vi "ep_Get Significance (ICM).vi"(0 "spectra points in window":T4(array[cluster]), 1 "pole pairs":i32, 2 "fundamental frequency [Hz]":dbl, 5 "peaks information":T3(array[cluster]), 7 "enough points for peak search?":bool[](array[boolean]), 9 "number of peaks":i32[](array[numeric]), 11 "error in (no error)":errorcluster, 12 "minimum max-magnitude":dbl, 13 "range of speed":T1) -> (4 "top3 speed data":cluster{"speed [RPM]":dbl, "slip":dbl}[](array[cluster]), 6 "top3 significance":dbl[](array[numeric]), 8 "top3 harmonic for speed calculation":T2[](array[typedef]), 14 "candidate speeds":cluster{"speed [RPM]":dbl, "slip":dbl}[](array[cluster]), 15 "error out":errorcluster)   [LabVIEW 2017]
uses:
  <vilib>/addons/Electrical Power/Motor Monitoring/subVIs/ep_Harmonic for Speed Calculation.ctl
  <vilib>/Analysis/baseanly.llb/Mean (DBL).vi
  <vilib>/Analysis/NI_AALBase.lvlib
  <vilib>/addons/Electrical Power/Motor Monitoring/NI_EP_Motor Monitoring.lvlib
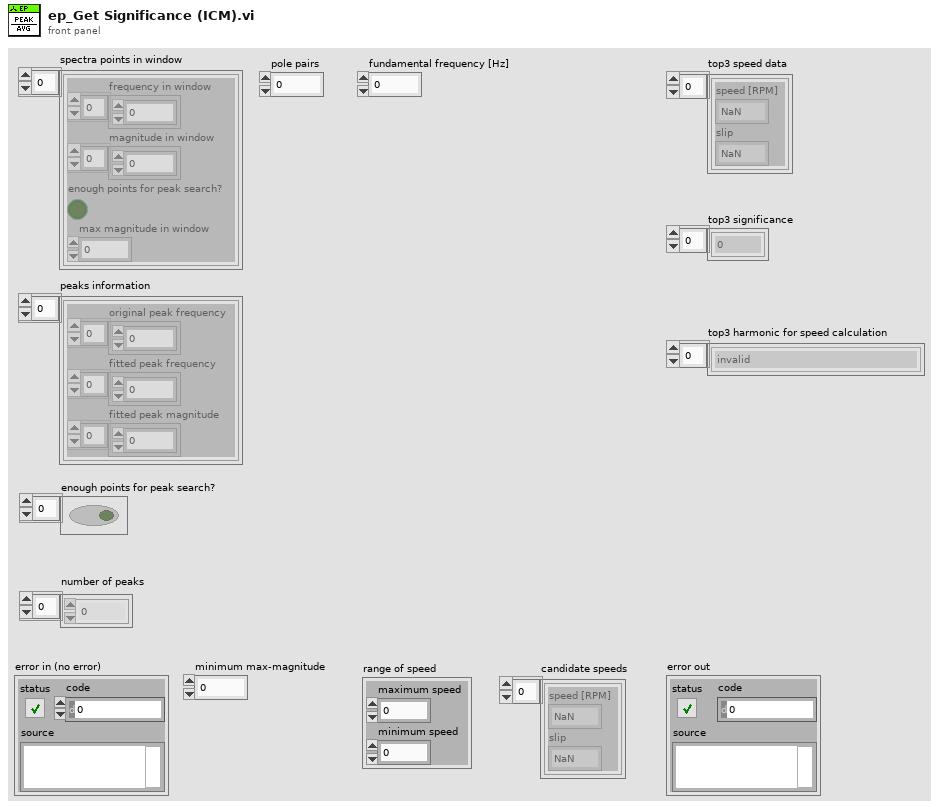
[diagram p1: front panel]
types:
  T1 = cluster{"maximum speed":dbl, "minimum speed":dbl}
  T2 = typedef "NI_EP_Motor Monitoring.lvlib/ep_Harmonic for Speed Calculation.ctl" = enum16{"invalid", "fr", "2fs-2fr", "2fs-fr", "2fr"}
  T3 = cluster{"original peak frequency":dbl[], "fitted peak frequency":dbl[], "fitted peak magnitude":dbl[]}[]
  T4 = cluster{"frequency in window":dbl[], "magnitude in window":dbl[], "enough points for peak search?":bool, "max magnitude in window":dbl}[]
  T5 = typedef "NI_EP_Motor Monitoring.lvlib/ep_Case for Speed Calculation.ctl" = enum16{"no available harmonic for speed calculation", "use the harmonic with highest magnitude", "use the harmonic with highest significance"}
  T6 = cluster{"frequency in window":dbl[], "magnitude in window":dbl[], "enough points for peak search?":bool, "max magnitude in window":dbl}
  T7 = cluster{"maximum frequency [Hz]":dbl, "slip error allowance":dbl, "minimum points for peak search":dbl, "accuracy of fs":dbl, "difference?":bool, " fs harmonics order":i32, "fs forbidden range":dbl, "p3:p1 valid significance ratio":dbl, "ratio for significance weighting":dbl, "significance weighting":dbl}
  T8 = cluster{"original peak frequency":dbl[], "fitted peak frequency":dbl[], "fitted peak magnitude":dbl[]}
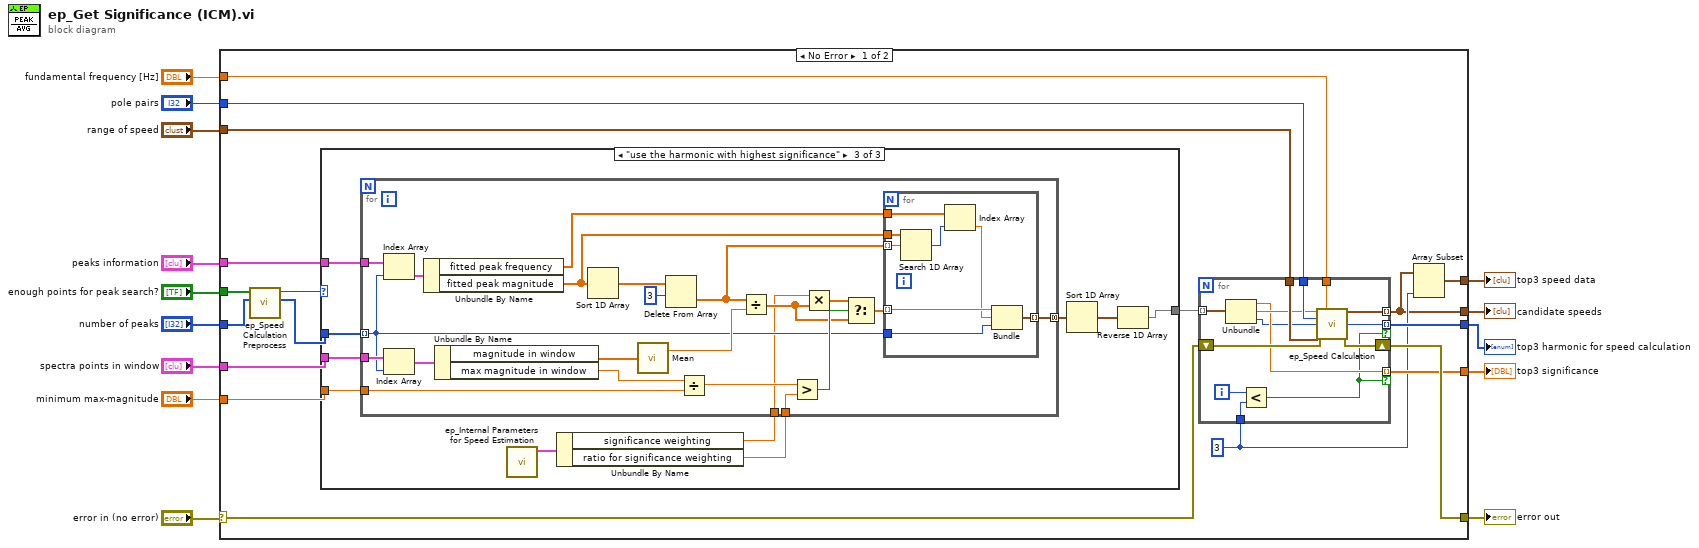
[diagram p0: block diagram]
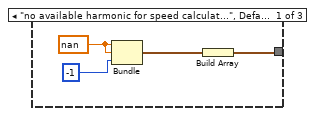
[diagram p2: hidden frame]
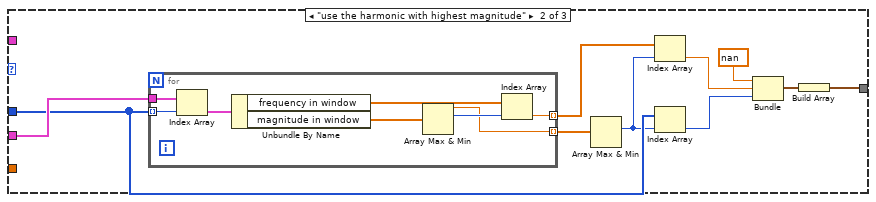
[diagram p3: hidden frame]
diagram:
  n1 = case shown="No Error" "error in (no error)" {
    selector: "error in (no error)" -> [w29 w109]
    tunnel: [w28 w109] -> w13
    tunnel: "peaks information" -> [w32 _]
    tunnel: "spectra points in window" -> [w30 _]
    tunnel: [w31 _] -> w10
    tunnel: [w16 _] -> w9
    tunnel: "fundamental frequency [Hz]" -> [w27 _]
    tunnel: "pole pairs" -> [w26 _]
    tunnel: "range of speed" -> [w25 _]
    tunnel: [w23 _] -> w5
    tunnel: "minimum max-magnitude" -> [w22 _]
    tunnel: "enough points for peak search?" -> [w19 _]
    tunnel: "number of peaks" -> [w18 _]
    tunnel: [w15 _] -> w1
    frame No Error {
      w17 = 3 ("y")
      n2 = call <vilib>:"ep_Speed Calculation Preprocess.vi"("number of peaks"=w18, "enough points for peak search?"=w19) -> ("harmonic for comparison"=w20:i32[], "case for speed calculation"=w21:T5)  [unwired: 8 in]
      n3 = case shown="\"use the harmonic with highest significance\"" w21 {
        tunnel: w32 -> [_ _ w78]
        tunnel: w30 -> [_ w60 w76]
        tunnel: w20 -> [_ w58 w77]
        tunnel: [w47 w54 w74] -> w24
        tunnel: w22 -> [_ _ w72]
        frame "no available harmonic for speed calculation", Default {
          w50 = nan
          n4 = Bundle(w50, w50, -1) -> (w48:cluster{dbl, dbl, i32})  [unwired: 1 in]
          n5 = Build Array(w48) -> (w47:cluster{dbl, dbl, i32}[])
        }
        frame "use the harmonic with highest magnitude" {
          n6 = for {
            tunnel: w58 -> [w67] mode=indexing
            tunnel: w60 -> [w68]
            tunnel: [w62] -> w59 mode=indexing
            tunnel: [w61] -> w57 mode=indexing
            n7 = Index Array(array=w68, index=w67) -> (element=w66:T6)
            n8 = Unbundle By Name(w66) -> ("frequency in window"=w64:dbl[], "magnitude in window"=w65:dbl[])
            n9 = Array Max & Min(array=w65) -> (max value=w62:dbl, max index (indices)=w63:i32)  [unwired: 2 out]
            n10 = Index Array(array=w64, index=w63) -> (element=w61:dbl)
          }
          n11 = Array Max & Min(array=w59) -> (max index (indices)=w56:i32)  [unwired: 3 out]
          n12 = Index Array(array=w57, index=w56) -> (element=w52:dbl)
          n13 = Index Array(array=w58, index=w56) -> (element=w51:i32)
          n14 = Bundle(nan, "frequency points"=w52, w51) -> (w53:cluster{dbl, "frequency points":dbl, i32})  [unwired: 1 in]
          n15 = Build Array(w53) -> (w54:cluster{dbl, "frequency points":dbl, i32}[])
        }
        frame "use the harmonic with highest significance" {
          n16 = call <vilib>:"ep_Internal Parameters for Speed Estimation.vi"() -> ("internal parameters for speed estimation"=w73:T7)  [unwired: 11 in]
          n17 = Unbundle By Name(w73) -> ("significance weighting"=w70:dbl, "ratio for significance weighting"=w71:dbl)
          n18 = for {
            tunnel: w78 -> [w100]
            tunnel: w77 -> [w87] mode=indexing
            tunnel: w76 -> [w97]
            tunnel: [w86] -> w75 mode=concatenating
            tunnel: w72 -> [w81]
            tunnel: w71 -> [w80]
            tunnel: w70 -> [w79]
            n19 = Index Array(array=w100, index=w87) -> (element=w98:T8)
            n20 = Index Array(array=w97, index=w87) -> (element=w92:T6)
            n21 = Unbundle By Name(w98) -> ("fitted peak frequency"=w99:dbl[], "fitted peak magnitude"=w96:dbl[])
            n22 = Unbundle By Name(w92) -> ("magnitude in window"=w91:dbl[], "max magnitude in window"=w82:dbl)
            n23 = Sort 1D Array(array=w96) -> (sorted array=w85:dbl[])
            n24 = call-poly <vilib>:"Mean.vi"("X"=w91) -> ("mean"=w93:dbl)  [unwired: 1 out]
            n25 = Delete From Array(array=w85, length=3 ("index")) -> (deleted portion=w83:dbl[])  [unwired: 1 in, 1 out]
            n26 = Divide(x=w82, y=w81) -> (x/y=w95:dbl)
            n27 = Divide(x=w83, y=w93) -> (x/y=w89:dbl[])
            n28 = Greater?(x=w95, y=w80) -> (0:w94:bool)
            n29 = Multiply(x=w79, y=w89) -> (x*y=w90:dbl[])
            n30 = Select(t=w90, s=w94, f=w89) -> (s? t:f=w88:dbl[])
            n31 = for {
              tunnel: w99 -> [w107]
              tunnel: w83 -> [w108] mode=indexing
              tunnel: w96 -> [w106]
              tunnel: w88 -> [w102] mode=indexing
              tunnel: w87 -> [w104]
              tunnel: [w103] -> w86 mode=indexing
              n32 = Search 1D Array(1D array=w106, element=w108) -> (index of element=w105:i32)  [unwired: 1 in]
              n33 = Index Array(array=w107, index=w105) -> (element=w101:dbl)
              n34 = Bundle(w102, w101, w104) -> (w103:cluster{dbl, dbl, i32})  [unwired: 1 in]
            }
          }
          n35 = Sort 1D Array(array=w75) -> (sorted array=w69:cluster{dbl, dbl, i32}[])
          n36 = Reverse 1D Array(array=w69) -> (reversed array=w74:cluster{dbl, dbl, i32}[])
        }
      }
      n37 = for {
        tunnel: [w36] -> w31 mode=indexing if=w34
        shift-right: [w45] -> w28
        shift-left: w29 -> [w46]
        tunnel: [w44] -> w15 mode=indexing
        tunnel: w27 -> [w43]
        tunnel: w26 -> [w42]
        tunnel: w25 -> [w41]
        tunnel: w24 -> [w40] mode=indexing
        tunnel: [w38] -> w23 mode=indexing if=w34
        tunnel: w17 -> [w33]
        i -> [w35]
        n38 = Unbundle(w40) -> (w38:dbl, "frequency points"=w39:dbl, w37:i32)
        n39 = Less?(x=w35, y=w33) -> (x < y?=w34:bool)
        n40 = call <vilib>:"ep_Speed Calculation.vi"("harmonic frequency"=w39, "fundamental frequency [Hz]"=w43, "pole pairs"=w42, "harmonic for speed calculation"=w37, "range of speed"=w41, "error in (no error)"=w46) -> ("speed data"=w44:cluster{"speed [RPM]":dbl, "slip":dbl}, "harmonic for speed calculation"=w36:T2, "error out"=w45:errorcluster)  [unwired: 7 in]
      }
      n41 = Array Subset(array=w15, length=w17) -> (w16:cluster{"speed [RPM]":dbl, "slip":dbl}[])  [unwired: 1 in]
    }
    frame Error {
    }
  }
  "error out" <- w13
  "top3 harmonic for speed calculation" <- w10
  "top3 significance" <- w5
  "top3 speed data" <- w9
  "candidate speeds" <- w1
